vi "stm test.vi"() -> ()   [LabVIEW 2017]
uses:
  <vilib>/Plasmionique/MB Master/MB_Master_Serial/MB_Master_Serial.lvclass
  D:/Program Files (x86)/National Instruments/LabVIEW 2017/vi.lib/Plasmionique/MB Master/MB_Master/MB_Master.lvclass
  <vilib>/Plasmionique/MB Master/MB Master.lvlib
panel:
  out "Registers":u16[](array[numeric])
  in  "stop":bool
  out "check local":bool[](array[boolean])
  out "local 1 wire error":bool[](array[boolean])
  out "fresh start":bool[](array[boolean])
  out "adres":u16[](array[numeric])
  out "wlacznik":bool[](array[boolean])
  out "blad":bool[](array[boolean])
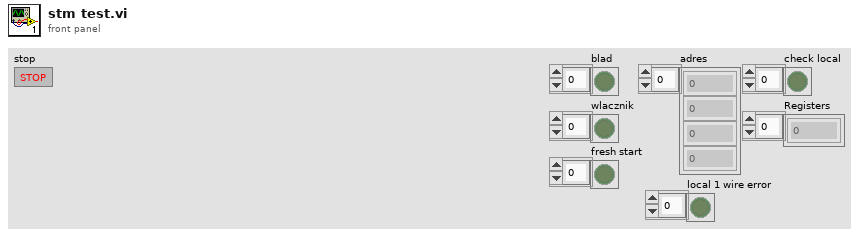
[diagram p1: front panel]
types:
  T1 = cluster{"baud rate (bps)":u32, "stop bits":u16, "parity":u16, "flow control":u16, "timeout":u32, "retries":i32}
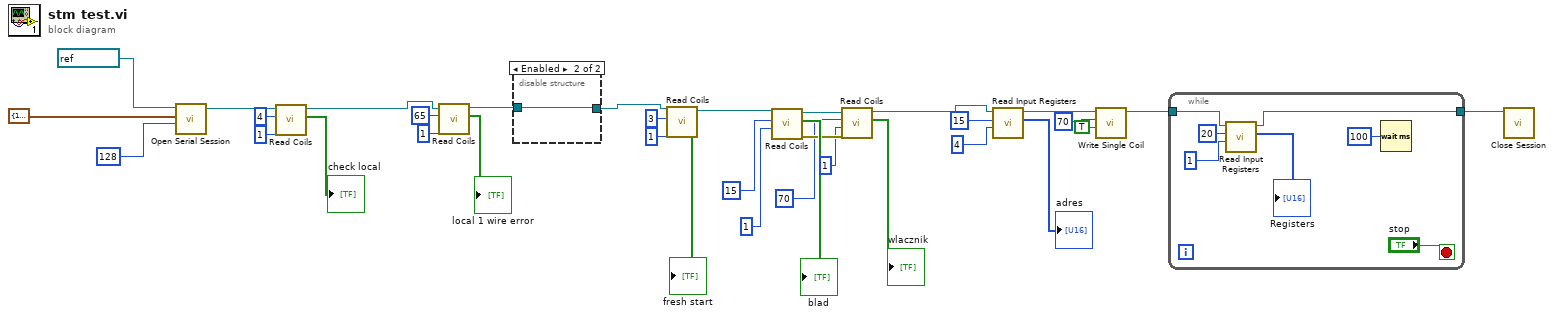
[diagram p0: block diagram]
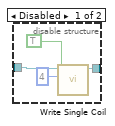
[diagram p2: hidden frame]
diagram:
  n1 = call <vilib>:"Open Serial Session.vi"("Slave ID"=u8 128, "Serial Config"=T1 {"baud rate (bps)"=19200, "stop bits"=10, "parity"=0, "flow control"=0, "timeout"=1000, "retries"=1}, "VISA Resource"=refnum<visa-resource-name> "COM6") -> ("MB_Serial session"=w14:refnum<class "MB_Master_Serial.lvclass">)  [unwired: 7 in, 1 out]
  n2 = call <vilib>:"Read Coils.vi"("quantity"=u16 1, "starting address"=u16 4, "MB session in"=w14) -> ("Coils"=→"check local":bool[], "MB session out"=w13:refnum<class "MB_Master_Serial.lvclass">)  [unwired: 6 in, 1 out]
  n3 = call <vilib>:"Read Coils.vi"("quantity"=u16 1, "starting address"=u16 65, "MB session in"=w13) -> ("Coils"=→"local 1 wire error":bool[], "MB session out"=w18:refnum<class "MB_Master_Serial.lvclass">)  [unwired: 6 in, 1 out]
  n4 = disable-structure shown="Enabled" {
    disable-tunnel: [w38 w39] -> w19
    disable-tunnel: w18 -> [w37 w39]
    frame Disabled {
      n5 = call <vilib>:"Write Single Coil.vi"("value"=TRUE, "address"=u16 4, "MB session in"=w37) -> ("MB session out"=w38:refnum<class "MB_Master_Serial.lvclass">)  [unwired: 7 in, 1 out]
    }
    frame Enabled {
    }
  }
  n6 = call <vilib>:"Read Coils.vi"("quantity"=u16 1, "starting address"=u16 3, "MB session in"=w19) -> ("Coils"=→"fresh start":bool[], "MB session out"=w23:refnum<class "MB_Master_Serial.lvclass">)  [unwired: 6 in, 1 out]
  n7 = call <vilib>:"Read Coils.vi"("quantity"=u16 1, "starting address"=u16 15, "MB session in"=w23) -> ("error out"=w27:errorcluster, "Coils"=→"blad":bool[], "MB session out"=w28:refnum<class "MB_Master_Serial.lvclass">)  [unwired: 6 in]
  n8 = call <vilib>:"Read Coils.vi"("error in (no error)"=w27, "quantity"=u16 1, "starting address"=u16 70, "MB session in"=w28) -> ("Coils"=→"wlacznik":bool[], "MB session out"=w8:refnum<class "MB_Master_Serial.lvclass">)  [unwired: 5 in, 1 out]
  n9 = call <vilib>:"Read Input Registers.vi"("quantity"=u16 4, "starting address"=u16 15, "MB session in"=w8) -> ("Registers"=→"adres":u16[], "MB session out"=w5:refnum<class "MB_Master_Serial.lvclass">)  [unwired: 6 in, 1 out]
  n10 = call <vilib>:"Write Single Coil.vi"("value"=TRUE, "address"=u16 70, "MB session in"=w5) -> ("MB session out"=w2:refnum<class "MB_Master_Serial.lvclass">)  [unwired: 7 in, 1 out]
  n11 = while {
    tunnel: w2 -> [w45]
    tunnel: [w41] -> w1
    stop <- "stop" stop-if-true
    n12 = call <vilib>:"Read Input Registers.vi"("quantity"=u16 1, "starting address"=u16 20, "MB session in"=w45) -> ("Registers"=→"Registers":u16[], "MB session out"=w41:refnum<class "MB_Master_Serial.lvclass">)  [unwired: 6 in, 1 out]
    n13 = Wait (ms)(milliseconds to wait=u32 100) -> ()  [unwired: 1 out]
  }
  n14 = call-dynamic "Close Session.vi"("MB_Serial session"=w1) -> ()  [unwired: 10 in, 1 out]
